vi "Unflatten Value.vi"(8 "error in (no error)":errorcluster, 10 "Value":string, 11 "Boolean in":refnum<class "String.lvclass">) -> (0 "error out":errorcluster, 3 "Boolean out":refnum<class "String.lvclass">)   [LabVIEW 2017, in "String.lvclass"]
uses:
  <vilib>/gpm_packages/@cs/data-type-serializer/source/String/String.lvclass
  <vilib>/gpm_packages/@cs/data-type-serializer/source/String/String.lvclass/String.ctl
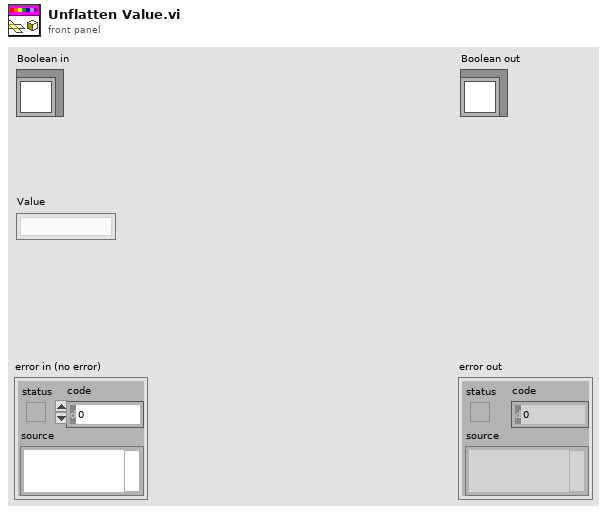
[diagram p1: front panel]
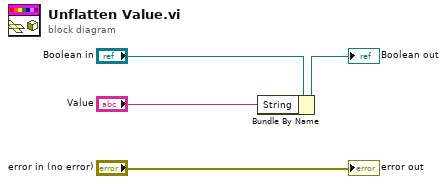
[diagram p0: block diagram]
diagram:
  n1 = Bundle By Name(cluster="Boolean in", "String"="Value") -> (→"Boolean out":refnum<class "String.lvclass">)
  "error out" <- "error in (no error)"
